vi "CSV_import_control_lasers_and_SMs_and_ICC4C_PROGRESS_ON_BUTTONCLICK.vi"() -> ()   [LabVIEW 2021]
uses:
  <vilib>/DAQmx/write.llb/DAQmx Write (Analog 1D DBL NChan 1Samp).vi
  <vilib>/DAQmx/create/channels.llb/DAQmx Create Channel (AO-Voltage-Basic).vi
  <vilib>/Utility/file.llb/Read Delimited Spreadsheet (DBL).vi
  <vilib>/DAQmx/miscellaneous.llb/DAQmx Fill In Error Info.vi
panel:
  in  "stop":bool
  in  "Inc":bool
  in  "ICC4C 3 (0-10V)":dbl
  in  "ICC4C 2 (0-10V)":dbl
  in  "ICC4C 1 (0-10V)":dbl
  in  "ICC4C 0 (0-10V)":dbl
  in  "Y2 (-10-10V)":dbl
  in  "X2 (-10-10V)":dbl
  in  "Continue Cycle?":bool
  out "Full Cycles":i32
  out "Phase I Iterations":i32
  out "Y1 (-10-10V)":dbl format="%_6g"
  out "X1 (-10-10V)":dbl format="%_6g"
  in  "Blanking (0-10v)":dbl=10.0
  in  "561 (0-10v)":dbl
  in  "514 (0-10v)":dbl
  in  "488 (0-10v)":dbl
  in  "445 (0-10v)":dbl
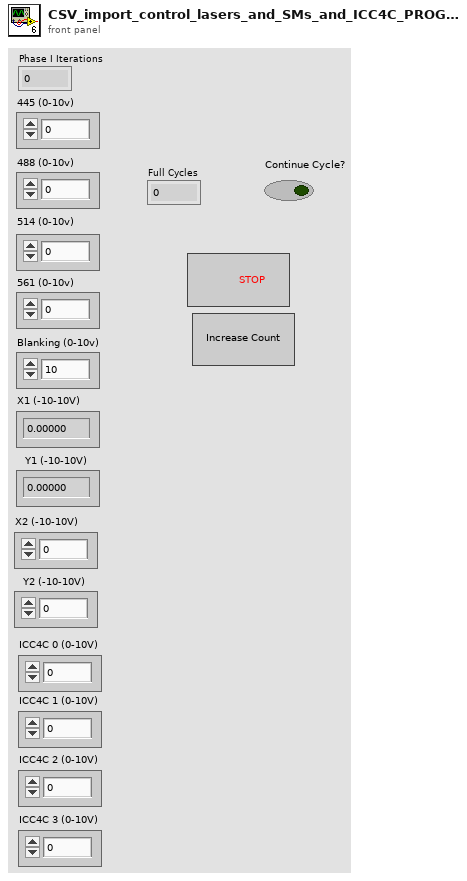
[diagram p1: front panel]
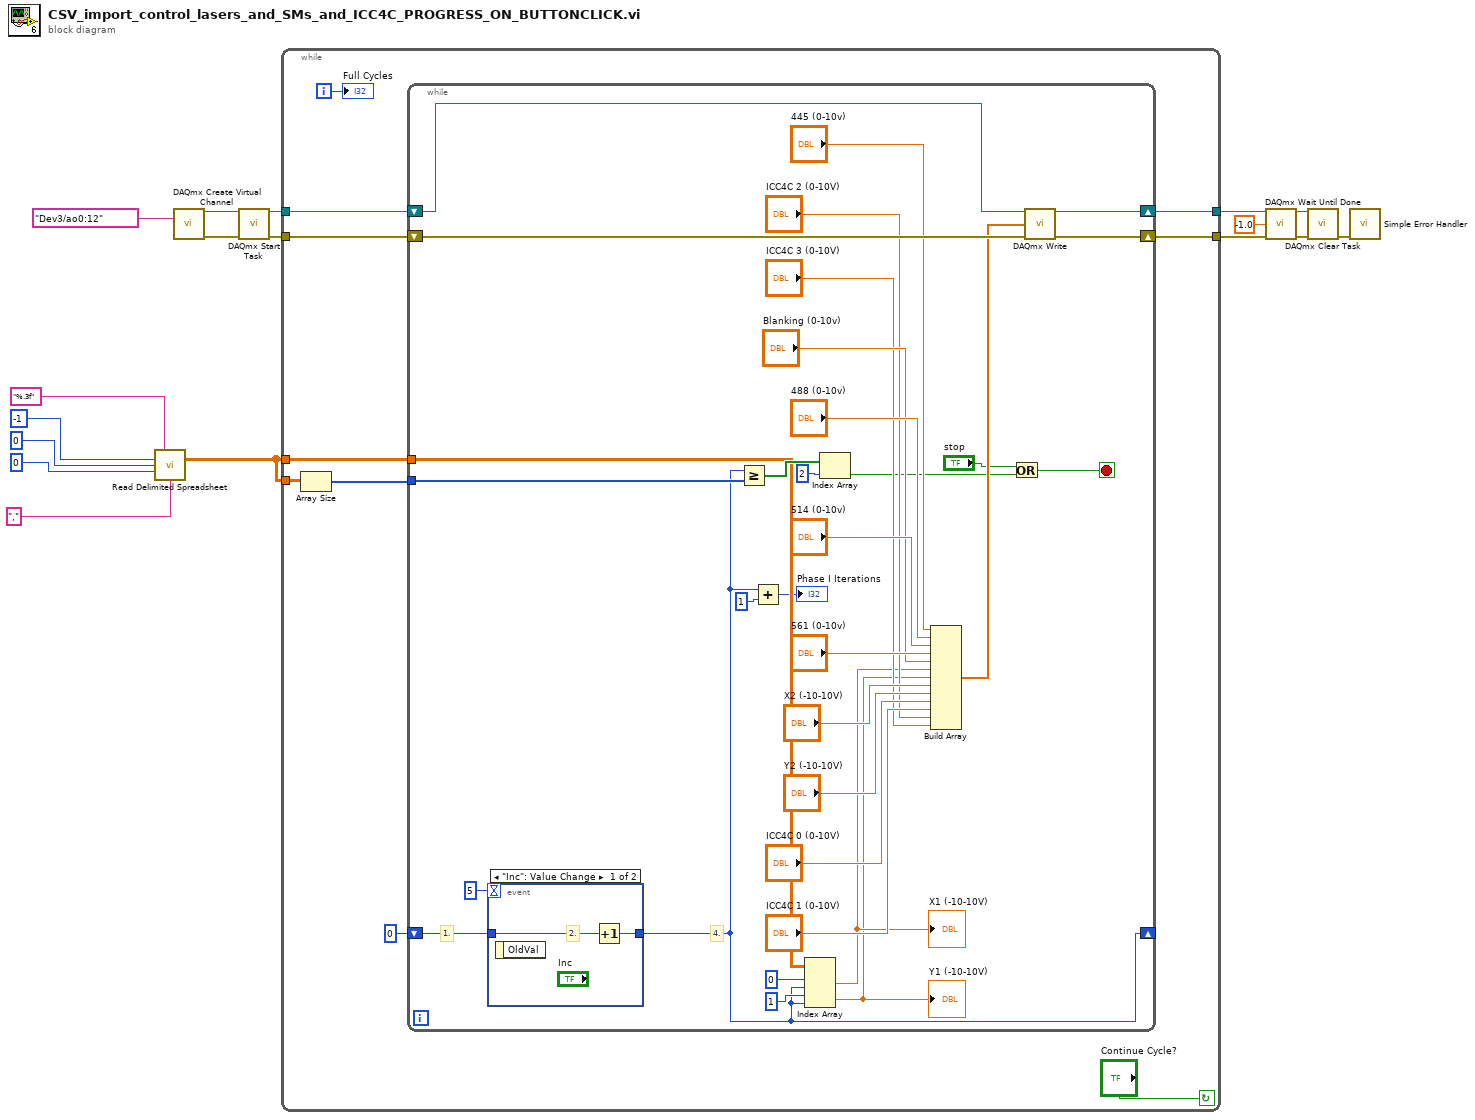
[diagram p0: block diagram]
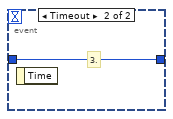
[diagram p2: hidden frame]
diagram:
  n1 = call-poly <vilib>:"Read Delimited Spreadsheet.vi"("format (%.3f)"="%.3f", "number of rows (all:-1)"=-1, "start of read offset (chars.:0)"=0, "max characters/row  (no limit:0)"=0, "delimiter (\\t)"=",") -> ("all rows"=w6:dbl[][])  [unwired: 5 in, 5 out]
  n2 = call-poly <vilib>:"DAQmx Create Virtual Channel.vi"("physical channels"=tag "Dev3/ao0:12") -> ("task out"=w10:refnum<k21>, "error out"=w9:errorcluster)  [unwired: 13 in]
  n3 = call <vilib>:"DAQmx Start Task.vi"("task/channels in"=w10, "error in"=w9) -> ("task out"=w8:refnum<k21>, "error out"=w7:errorcluster)  [unwired: 12 in]
  n4 = while {
    tunnel: [w23] -> w13
    tunnel: [w22] -> w12
    tunnel: w8 -> [w26]
    tunnel: w7 -> [w25]
    tunnel: w6 -> [w20]
    tunnel: w6 -> [w19]
    i -> [w27]
    stop <- "Continue Cycle?" continue-if-true
    n5 = Array Size(array=w20) -> (size(s)=w21:i32[])
    n6 = while {
      shift-right: [w57] -> w23
      shift-left: w26 -> [w59]
      shift-right: [w56] -> w22
      shift-left: w25 -> [w58]
      tunnel: w21 -> [w42]
      tunnel: w19 -> [w39]
      shift-right: [w30] -> _
      shift-left: 0 -> [w34]
      stop <- w31 stop-if-true
      # "4."
      # "1."
      n7 = event shown="[0] \"Inc\": Value Change" {
        selector: _ -> [_ _]
        dyn-events: _ -> [_ _]
        timeout: 5 -> [_ _]
        tunnel: w34 -> [w61 w62]
        tunnel: [w60 w62] -> w30
        event "Inc": Value Change {
          # "2."
          n8 = event-data() -> ()  [unwired: 2 out]
          n9 = Increment(x=w61) -> (x+1=w60:i32)
        }
        event Timeout {
          # "3."
          n10 = event-data() -> ()  [unwired: 2 out]
        }
      }
      n11 = Greater Or Equal?(x=w30, y=w42) -> (x >= y?=w41:bool[])
      n12 = Add(x=w30, y=1) -> (x+y=→"Phase I Iterations":i32)
      n13 = Index Array(array=w39, index (row) #1=0, index (col) #1=w30, index (row) #2=1, index (col) #2=w30) -> (element #1=w43:dbl, element #2=w38:dbl)
      "X1 (-10-10V)" <- w43
      "Y1 (-10-10V)" <- w38
      n14 = Index Array(array=w41, index=2) -> (element=w32:bool)
      n15 = Build Array("445 (0-10v)", "488 (0-10v)", "514 (0-10v)", "561 (0-10v)", "Blanking (0-10v)", w43, w38, "X2 (-10-10V)", "Y2 (-10-10V)", "ICC4C 0 (0-10V)", "ICC4C 1 (0-10V)", "ICC4C 2 (0-10V)", "ICC4C 3 (0-10V)") -> (w55:dbl[])
      n16 = Or(x="stop", y=w32) -> (x .or. y?=w31:bool)
      n17 = call-poly <vilib>:"DAQmx Write.vi"("task/channels in"=w59, "data"=w55, "error in"=w58) -> ("task out"=w57:refnum<k21>, "error out"=w56:errorcluster)  [unwired: 10 in, 1 out]
    }
    "Full Cycles" <- w27
  }
  n18 = call <vilib>:"DAQmx Wait Until Done.vi"("task/channels in"=w13, "timeout (sec)"=-1.0, "error in"=w12) -> ("task out"=w16:refnum<k21>, "error out"=w15:errorcluster)  [unwired: 11 in]
  n19 = call <vilib>:"DAQmx Clear Task.vi"("task in"=w16, "error in"=w15) -> ("error out"=w17:errorcluster)  [unwired: 13 in]
  n20 = call <vilib>:"Simple Error Handler.vi"("error in (no error)"=w17) -> ()  [unwired: 4 in, 5 out]
